vi "WritePressureToReport.vi"(8 "error in (no error)":errorcluster, 9 "LowPressure":bool, 10 "Initial":bool) -> (0 "error out":errorcluster)   [LabVIEW 2018, in "S5.lvclass"]
uses:
  S5.lvclass
  Public Controls/ReportHeader.ctl
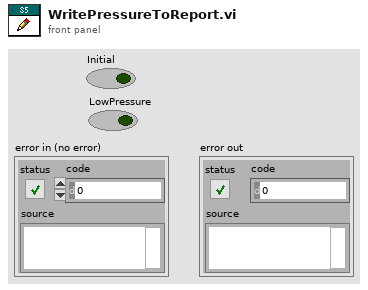
[diagram p1: front panel]
types:
  T1 = typedef "S5.lvclass/ReportHeader.ctl" = string
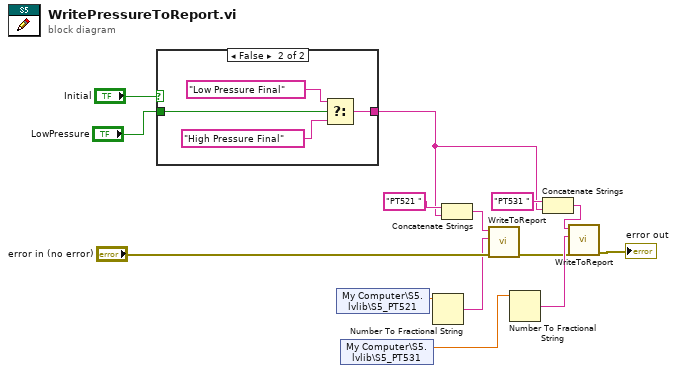
[diagram p0: block diagram]
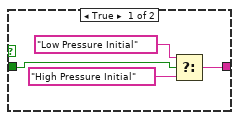
[diagram p2: hidden frame]
diagram:
  n1 = case shown="False" "Initial" {
    tunnel: "LowPressure" -> [w16 w22]
    tunnel: [w15 w19] -> w2
    frame True {
      n2 = Select(t=T1 "Low Pressure Initial" ("Header"), s=w16, f=T1 "High Pressure Initial" ("Header")) -> (s? t:f=w15:T1)
    }
    frame False {
      n3 = Select(t=T1 "Low Pressure Final" ("Header"), s=w22, f=T1 "High Pressure Final" ("Header")) -> (s? t:f=w19:T1)
    }
  }
  n4 = shared-variable "My Computer\\S5.lvlib\\S5_PT521"() -> (w11:dbl)  [unwired: 1 in, 1 out]
  n5 = shared-variable "My Computer\\S5.lvlib\\S5_PT531"() -> (w9:dbl)  [unwired: 1 in, 1 out]
  n6 = Number To Fractional String(number=w11) -> (F-format string=w10:string)  [unwired: 3 in]
  n7 = Concatenate Strings("PT521 " ("string"), w2) -> (w6:string)
  n8 = call "WriteToReport.vi"("error in"="error in (no error)", "Value"=w10, "Header"=w6) -> ("error out"=w7:errorcluster)  [unwired: 8 in]
  n9 = Number To Fractional String(number=w9) -> (F-format string=w8:string)  [unwired: 3 in]
  n10 = Concatenate Strings("PT531 " ("string"), w2) -> (w3:string)
  n11 = call "WriteToReport.vi"("error in"=w7, "Value"=w8, "Header"=w3) -> ("error out"=→"error out":errorcluster)  [unwired: 8 in]
